vi "Test_DeleteItem_NotInTable_NotFound.vi"(8 "error in (no error)":errorcluster, 11 "TestCase in":refnum<class "TestComposedLookupTable.lvclass">) -> (0 "error out":errorcluster, 3 "TestCase out":refnum<class "TestComposedLookupTable.lvclass">)   [LabVIEW 2017, in "TestComposedLookupTable.lvclass"]
uses:
  TestComposedLookupTable.lvclass
  Source/LookupTable/LookupTable.lvclass/LookupTable.ctl
  b0d92e1d-d4a4-4958-9cd7-a9a25488efb3.vi
  Source/LookupTable/Read Table Reference.vi
  Source/LookupTable/LookupTable.lvclass
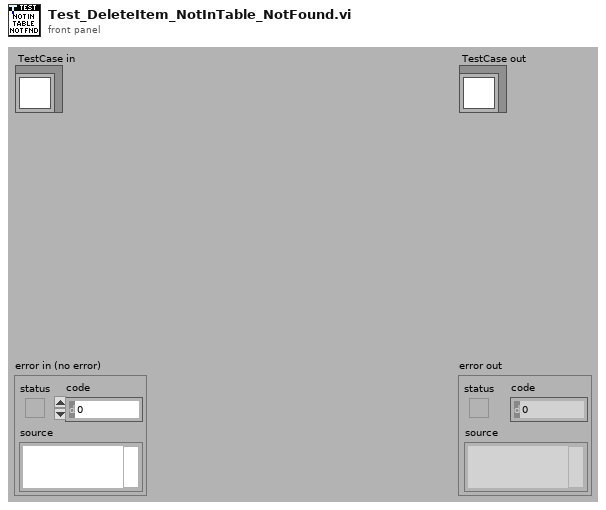
[diagram p1: front panel]
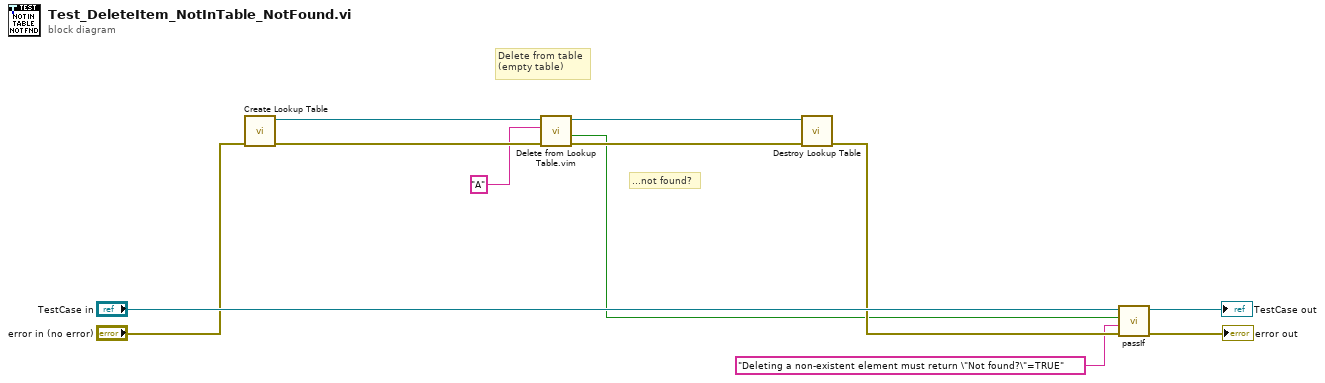
[diagram p0: block diagram]
diagram:
  # "...not found?"
  # "Delete from table\n(empty table)"
  n1 = call "Create Lookup Table.vi"("error in (no error)"="error in (no error)") -> ("error out"=w12:errorcluster, "LookupTable Reference"=w8:refnum<data-value>)  [unwired: 9 in]
  n2 = call "Delete from Lookup Table.vim"("error in (no error)"=w12, "Item Name"="A", "LookupTable Reference"=w8) -> ("error out"=w5:errorcluster, "Not Found?"=w2:bool, "LookupTable Reference Out"=w4:refnum<data-value>)  [unwired: 6 in]
  n3 = call "Destroy Lookup Table.vi"("error in (no error)"=w5, "LookupTable Reference"=w4) -> ("error out"=w6:errorcluster)  [unwired: 9 in]
  n4 = call-dynamic "passIf.vi"("error in (no error)"=w6, "message (\"\")"="Deleting a non-existent element must return \"Not found?\"=TRUE" ("message (\"\")"), "pass"=w2, "TestCase in"="TestCase in") -> ("error out"=→"error out":errorcluster, "TestCase out"=→"TestCase out":refnum<class "TestComposedLookupTable.lvclass">)  [unwired: 6 in]
